vi "DAQ_pressure_flow_subVI_V2.vi"(0 "vac press":dbl[](array[numeric])) -> (3 "read pressure":dbl, 6 "read vapor flow":dbl, 10 "press/RH/gas/vapor":T1, 15 "read gas flow":dbl)   [LabVIEW 2014]
panel:
  out "read RH":string
  out "save pressure":string
  out "save gas flow":string
  out "save vapor flow":string
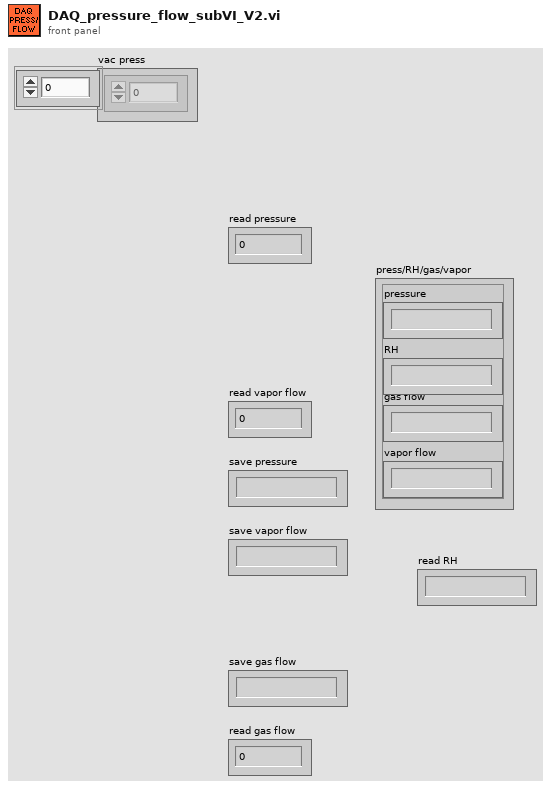
[diagram p1: front panel]
types:
  T1 = cluster{"pressure":string, "RH":string, "gas flow":string, "vapor flow":string}
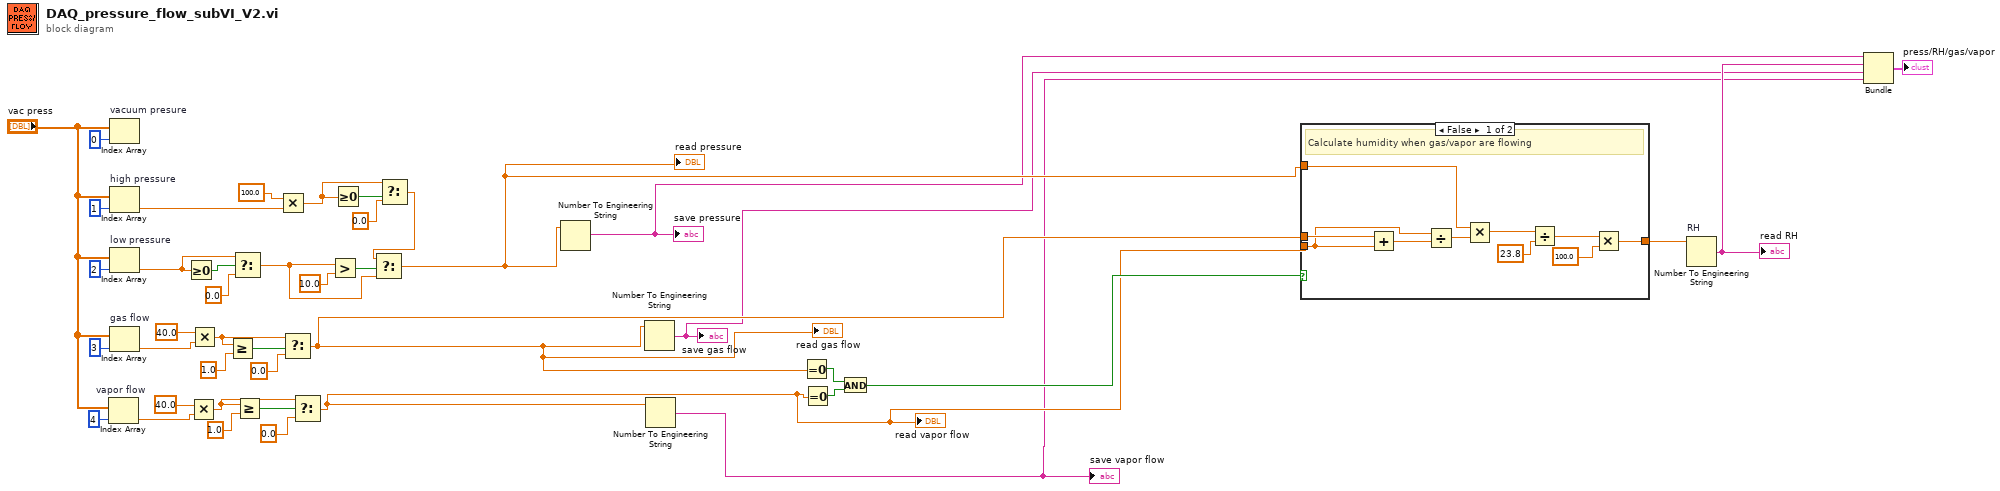
[diagram p0: block diagram]
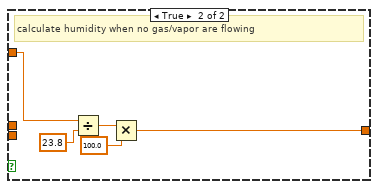
[diagram p2: hidden frame]
diagram:
  n1 = Index Array "vapor flow"(array="vac press", index=4) -> (element=w22:dbl)
  n2 = Index Array "vacuum presure"(array="vac press", index=0) -> ()  [unwired: 1 out]
  n3 = Index Array "high pressure"(array="vac press", index=1) -> (element=w15:dbl)
  n4 = Index Array "low pressure"(array="vac press", index=2) -> (element=w38:dbl)
  n5 = Index Array "gas flow"(array="vac press", index=3) -> (element=w20:dbl)
  n6 = Greater Or Equal To 0?(x=w38) -> (x >= 0?=w37:bool)
  n7 = Multiply(x=40.0, y=w22) -> (x*y=w29:dbl)
  n8 = Multiply(x=40.0, y=w20) -> (x*y=w32:dbl)
  n9 = Greater Or Equal?(x=w32, y=1.0) -> (x >= y?=w33:bool)
  n10 = Select(t=w38, s=w37, f=0.0) -> (s? t:f=w39:dbl)
  n11 = Greater Or Equal?(x=w29, y=1.0) -> (x >= y?=w30:bool)
  n12 = Multiply(x=100.0, y=w15) -> (x*y=w27:dbl)
  n13 = Select(t=w32, s=w33, f=0.0) -> (s? t:f=w6:dbl)
  "read gas flow" <- w6
  n14 = Select(t=w29, s=w30, f=0.0) -> (s? t:f=w7:dbl)
  "read vapor flow" <- w7
  n15 = Greater?(x=w39, y=10.0) -> (0:w34:bool)
  n16 = Greater Or Equal To 0?(x=w27) -> (x >= 0?=w25:bool)
  n17 = Select(t=w27, s=w25, f=0.0) -> (s? t:f=w35:dbl)
  n18 = Select(t=w35, s=w34, f=w39) -> (s? t:f=w9:dbl)
  "read pressure" <- w9
  n19 = Number To Engineering String(4:w9) -> (0:w5:string)  [unwired: 3 in]
  "save pressure" <- w5
  n20 = Number To Engineering String(4:w6) -> (0:w3:string)  [unwired: 3 in]
  "save gas flow" <- w3
  n21 = Number To Engineering String(4:w7) -> (0:w2:string)  [unwired: 3 in]
  "save vapor flow" <- w2
  n22 = Equal To 0?(x=w6) -> (x = 0?=w42:bool)
  n23 = Equal To 0?(x=w7) -> (x = 0?=w41:bool)
  n24 = And(x=w42, y=w41) -> (x .and. y?=w8:bool)
  n25 = case shown="False" w8 {
    tunnel: w9 -> [w44 w54]
    tunnel: [w43 w53] -> w10
    tunnel: w6 -> [w52 _]
    tunnel: w7 -> [w50 _]
    frame False {
      # "Calculate humidity when gas/vapor are flowing"
      n26 = Add(x=w52, y=w50) -> (x+y=w51:dbl)
      n27 = Divide(x=w50, y=w51) -> (x/y=w45:dbl)
      n28 = Multiply(x=w44, y=w45) -> (x*y=w46:dbl)
      n29 = Divide(x=w46, y=23.8) -> (x/y=w48:dbl)
      n30 = Multiply(x=w48, y=100.0) -> (x*y=w43:dbl)
    }
    frame True {
      # "calculate humidity when no gas/vapor are flowing"
      n31 = Divide(x=w54, y=23.8) -> (x/y=w56:dbl)
      n32 = Multiply(x=w56, y=100.0) -> (x*y=w53:dbl)
    }
  }
  n33 = Number To Engineering String "RH"(4:w10) -> (0:w4:string)  [unwired: 3 in]
  "read RH" <- w4
  n34 = Bundle(w5, w4, w3, w2) -> (→"press/RH/gas/vapor":cluster{string, string, string, string})  [unwired: 1 in]
